vi "Display.vi"(0 "Results":dbl[][](array[numeric])=[[0.09977187633195997, -0.006203643047489001, 0.09996455619021995, -3.557972183798793], [0.29923081468669355, -0.01860728479310232, 0.29980879157463614, -3.5582829459211704], [0.29923081468669355, -0.01860728479310232, 0.29980879157463614, -3.5582829459211704], [0.29923081468669355, -0.01860728479310232, 0.29980879157463614, -3.5582829459211704]], 2 "Display":u16(ring) items=["X and Y", "R and Theta"], 3 "Lock-in #":u16(ring) items=["Lock-in #1", "Lock-in #2", "Lock-in #3", "Lock-in #4"], 5 "Amplifier Settings":u16[](array[ring])=[0, 1, 2, 3] items=["DLPCA1", "DLPCA2", "DLPVA3", "DLPVA4"]) -> (6 "Display 1":string=" 144.059967   mV", 7 "Display 2":string=" 144.059967   mV", 9 "Array":dbl[](array[numeric]), 10 "Array 2":dbl[](array[numeric]))   [LabVIEW 2013, in "Lock-In Variable Channels_2.lvclass"]
uses:
  Variable Channel O.O.P/Lock-In Variable Channels_2.lvclass
panel:
  out "n":dbl
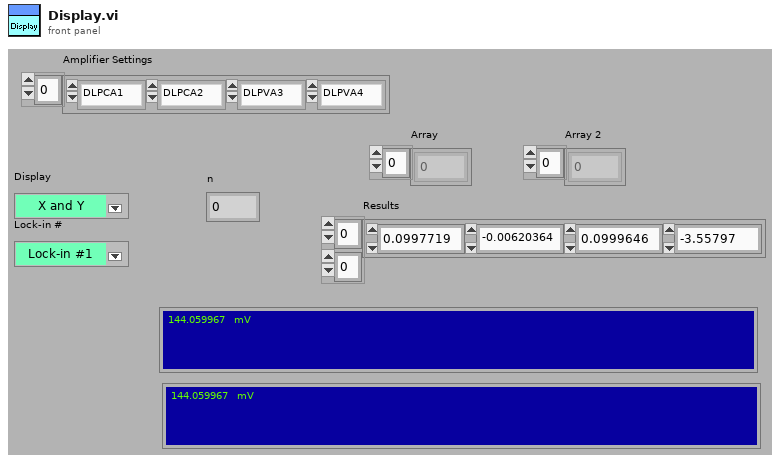
[diagram p1: front panel]
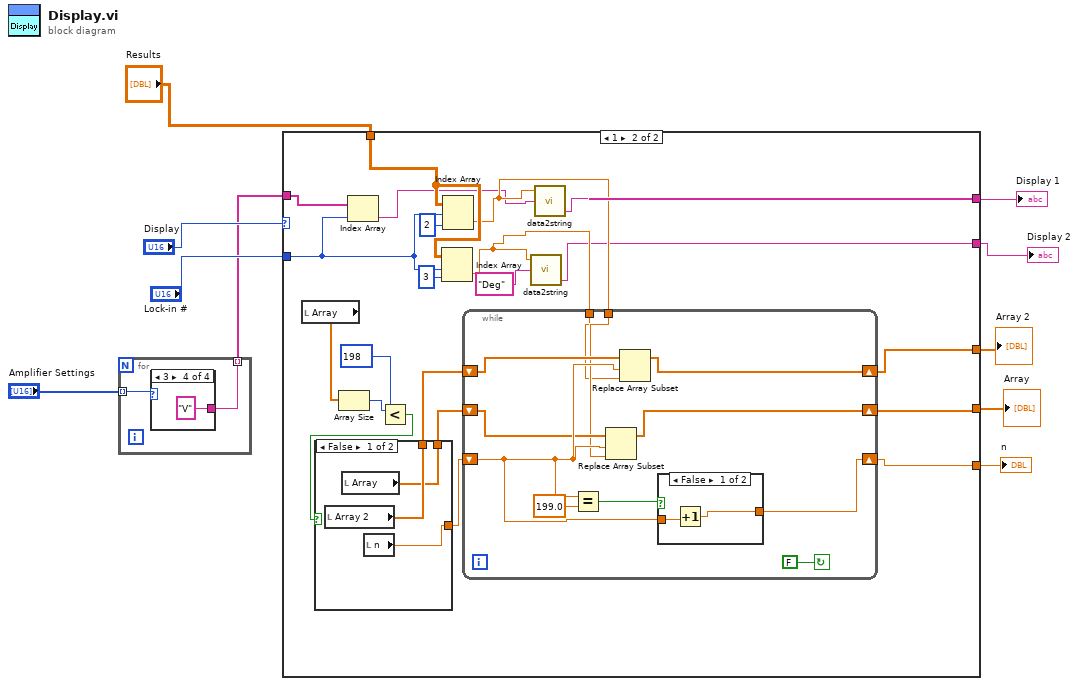
[diagram p0: block diagram]
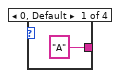
[diagram p2: hidden frame]
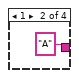
[diagram p3: hidden frame]
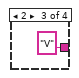
[diagram p4: hidden frame]
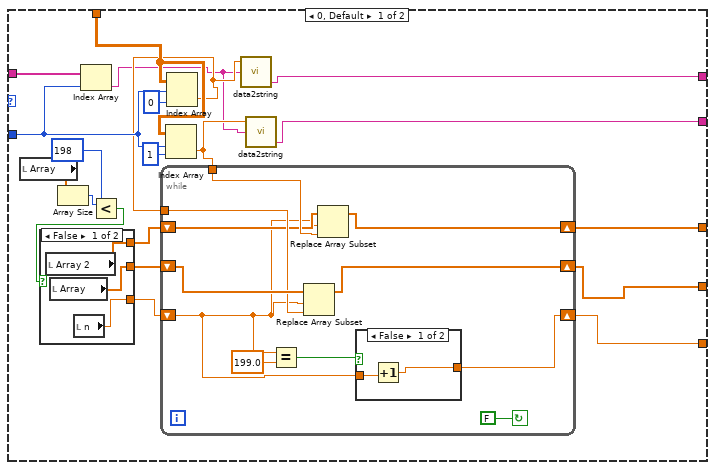
[diagram p5: hidden frame]
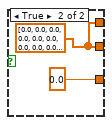
[diagram p6: hidden frame]
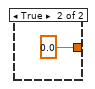
[diagram p7: hidden frame]
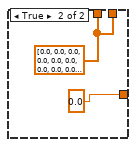
[diagram p8: hidden frame]
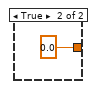
[diagram p9: hidden frame]
diagram:
  n1 = for {
    tunnel: "Amplifier Settings" -> [w12] mode=indexing
    tunnel: [w11] -> w1 mode=indexing
    n2 = case shown="3" w12 {
      tunnel: ["A" ("Units") "A" ("Units") "V" ("Units") "V" ("Units")] -> w11
      frame 0, Default {
      }
      frame 1 {
      }
      frame 2 {
      }
      frame 3 {
      }
    }
  }
  n3 = case shown="1" "Display" {
    tunnel: "Results" -> [w35 w74]
    tunnel: [w20 w59] -> w8
    tunnel: [w17 w56] -> w9
    tunnel: "Lock-in #" -> [w22 w62]
    tunnel: [w26 w68] -> w5
    tunnel: [w25 w67] -> w4
    tunnel: [w24 w65] -> w3
    tunnel: w1 -> [w23 w63]
    frame 0, Default {
      n4 = local read "Array"() -> (w31:dbl[])
      n5 = Array Size(array=w31) -> (size(s)=w30:i32)
      n6 = Index Array(array=w23, index=w22) -> (element=w18:string)
      n7 = Less?(x=w30, y=198) -> (x < y?=w28:bool)
      n8 = case shown="False" w28 {
        tunnel: [w38 w40] -> w33
        tunnel: [w39 0.0 ("y")] -> w32
        tunnel: [w37 w40] -> w27
        frame False {
          n9 = local read "Array 2"() -> (w37:dbl[])
          n10 = local read "Array"() -> (w38:dbl[])
          n11 = local read "n"() -> (w39:dbl)
        }
        frame True {
          w40 = dbl[] [0.0, 0.0, 0.0, 0.0, 0.0, 0.0, 0.0, 0.0, 0.0, 0.0, 0.0, 0.0, 0.0, 0.0, 0.0, 0.0, 0.0, 0.0, 0.0, 0.0, 0.0, 0.0, 0.0, 0.0, 0.0, 0.0, 0.0, 0.0, 0.0, 0.0, 0.0, 0.0, 0.0, 0.0, 0.0, 0.0, 0.0, 0.0, 0.0, 0.0, 0.0, 0.0, 0.0, 0.0, 0.0, 0.0, 0.0, 0.0, 0.0, 0.0, 0.0, 0.0, 0.0, 0.0, 0.0, 0.0, 0.0, 0.0, 0.0, 0.0, 0.0, 0.0, 0.0, 0.0, 0.0, 0.0, 0.0, 0.0, 0.0, 0.0, 0.0, 0.0, 0.0, 0.0, 0.0, 0.0, 0.0, 0.0, 0.0, 0.0, 0.0, 0.0, 0.0, 0.0, 0.0, 0.0, 0.0, 0.0, 0.0, 0.0, 0.0, 0.0, 0.0, 0.0, 0.0, 0.0, 0.0, 0.0, 0.0, 0.0, 0.0, 0.0, 0.0, 0.0, 0.0, 0.0, 0.0, 0.0, 0.0, 0.0, 0.0, 0.0, 0.0, 0.0, 0.0, 0.0, 0.0, 0.0, 0.0, 0.0, 0.0, 0.0, 0.0, 0.0, 0.0, 0.0, 0.0, 0.0, 0.0, 0.0, 0.0, 0.0, 0.0, 0.0, 0.0, 0.0, 0.0, 0.0, 0.0, 0.0, 0.0, 0.0, 0.0, 0.0, 0.0, 0.0, 0.0, 0.0, 0.0, 0.0, 0.0, 0.0, 0.0, 0.0, 0.0, 0.0, 0.0, 0.0, 0.0, 0.0, 0.0, 0.0, 0.0, 0.0, 0.0, 0.0, 0.0, 0.0, 0.0, 0.0, 0.0, 0.0, 0.0, 0.0, 0.0, 0.0, 0.0, 0.0, 0.0, 0.0, 0.0, 0.0, 0.0, 0.0, 0.0, 0.0, 0.0, 0.0, 0.0, 0.0, 0.0, 0.0, 0.0, 0.0, 0.0, 0.0, 0.0, 0.0, 0.0, 0.0]
        }
      }
      n12 = Index Array(array=w35, index (row)=w22, index (col)=1 ("disabled index (col)")) -> (element=w19:dbl)
      n13 = Index Array(array=w35, index (row)=w22, index (col)=0 ("disabled index (col)")) -> (element=w21:dbl)
      n14 = while {
        tunnel: w21 -> [w50]
        shift-right: [w49] -> w25
        shift-left: w33 -> [w51]
        shift-right: [w46] -> w24
        shift-left: w32 -> [w42]
        tunnel: w19 -> [w45]
        shift-right: [w44] -> w26
        shift-left: w27 -> [w43]
        stop <- FALSE continue-if-true
        n15 = Equal?(x=w42, y=199.0) -> (x = y?=w47:bool)
        n16 = Replace Array Subset(array=w51, new element=w50, index=w42) -> (w49:dbl[])
        n17 = Replace Array Subset(array=w43, new element=w45, index=w42) -> (w44:dbl[])
        n18 = case shown="False" w47 {
          tunnel: [w53 0.0 ("y")] -> w46
          tunnel: w42 -> [w54 _]
          frame False {
            n19 = Increment(x=w54) -> (x+1=w53:dbl)
          }
          frame True {
          }
        }
      }
      n20 = call "data2string.vi"("Units"=w18, "Numeric"=w21) -> ("resulting string"=w20:string)
      n21 = call "data2string.vi"("Units"=w18, "Numeric"=w19) -> ("resulting string"=w17:string)
    }
    frame 1 {
      n22 = local read "Array"() -> (w64:dbl[])
      n23 = Array Size(array=w64) -> (size(s)=w72:i32)
      n24 = Index Array(array=w63, index=w62) -> (element=w60:string)
      n25 = Less?(x=w72, y=198) -> (x < y?=w71:bool)
      n26 = case shown="False" w71 {
        tunnel: [w79 w81] -> w70
        tunnel: [w78 w81] -> w69
        tunnel: [w77 0.0 ("y")] -> w66
        frame False {
          n27 = local read "Array 2"() -> (w79:dbl[])
          n28 = local read "Array"() -> (w78:dbl[])
          n29 = local read "n"() -> (w77:dbl)
        }
        frame True {
          w81 = dbl[] [0.0, 0.0, 0.0, 0.0, 0.0, 0.0, 0.0, 0.0, 0.0, 0.0, 0.0, 0.0, 0.0, 0.0, 0.0, 0.0, 0.0, 0.0, 0.0, 0.0, 0.0, 0.0, 0.0, 0.0, 0.0, 0.0, 0.0, 0.0, 0.0, 0.0, 0.0, 0.0, 0.0, 0.0, 0.0, 0.0, 0.0, 0.0, 0.0, 0.0, 0.0, 0.0, 0.0, 0.0, 0.0, 0.0, 0.0, 0.0, 0.0, 0.0, 0.0, 0.0, 0.0, 0.0, 0.0, 0.0, 0.0, 0.0, 0.0, 0.0, 0.0, 0.0, 0.0, 0.0, 0.0, 0.0, 0.0, 0.0, 0.0, 0.0, 0.0, 0.0, 0.0, 0.0, 0.0, 0.0, 0.0, 0.0, 0.0, 0.0, 0.0, 0.0, 0.0, 0.0, 0.0, 0.0, 0.0, 0.0, 0.0, 0.0, 0.0, 0.0, 0.0, 0.0, 0.0, 0.0, 0.0, 0.0, 0.0, 0.0, 0.0, 0.0, 0.0, 0.0, 0.0, 0.0, 0.0, 0.0, 0.0, 0.0, 0.0, 0.0, 0.0, 0.0, 0.0, 0.0, 0.0, 0.0, 0.0, 0.0, 0.0, 0.0, 0.0, 0.0, 0.0, 0.0, 0.0, 0.0, 0.0, 0.0, 0.0, 0.0, 0.0, 0.0, 0.0, 0.0, 0.0, 0.0, 0.0, 0.0, 0.0, 0.0, 0.0, 0.0, 0.0, 0.0, 0.0, 0.0, 0.0, 0.0, 0.0, 0.0, 0.0, 0.0, 0.0, 0.0, 0.0, 0.0, 0.0, 0.0, 0.0, 0.0, 0.0, 0.0, 0.0, 0.0, 0.0, 0.0, 0.0, 0.0, 0.0, 0.0, 0.0, 0.0, 0.0, 0.0, 0.0, 0.0, 0.0, 0.0, 0.0, 0.0, 0.0, 0.0, 0.0, 0.0, 0.0, 0.0, 0.0, 0.0, 0.0, 0.0, 0.0, 0.0, 0.0, 0.0, 0.0, 0.0, 0.0, 0.0]
        }
      }
      n30 = Index Array(array=w74, index (row)=w62, index (col)=3 ("disabled index (col)")) -> (element=w58:dbl)
      n31 = Index Array(array=w74, index (row)=w62, index (col)=2 ("disabled index (col)")) -> (element=w61:dbl)
      n32 = while {
        shift-right: [w91] -> w67
        shift-left: w69 -> [w84]
        shift-right: [w88] -> w65
        shift-left: w66 -> [w87]
        shift-right: [w86] -> w68
        shift-left: w70 -> [w85]
        tunnel: w61 -> [w83]
        tunnel: w58 -> [w82]
        stop <- FALSE continue-if-true
        n33 = Equal?(x=w87, y=199.0) -> (x = y?=w89:bool)
        n34 = Replace Array Subset(array=w84, new element=w83, index=w87) -> (w91:dbl[])
        n35 = Replace Array Subset(array=w85, new element=w82, index=w87) -> (w86:dbl[])
        n36 = case shown="False" w89 {
          tunnel: [w93 0.0 ("y")] -> w88
          tunnel: w87 -> [w94 _]
          frame False {
            n37 = Increment(x=w94) -> (x+1=w93:dbl)
          }
          frame True {
          }
        }
      }
      n38 = call "data2string.vi"("Units"="Deg", "Numeric"=w58) -> ("resulting string"=w56:string)
      n39 = call "data2string.vi"("Units"=w60, "Numeric"=w61) -> ("resulting string"=w59:string)
    }
  }
  "Display 2" <- w9
  "Display 1" <- w8
  "Array 2" <- w5
  "Array" <- w4
  "n" <- w3
